vi "Initialize TX Transfer.vi"(7 "component name":string, 8 "error in":errorcluster, 9 "timeout (ms)":i32=1000 format="%.0f ms", 11 "Transfer Configuration in":refnum<class "Transfer Configuration.lvclass">) -> (0 "error out":errorcluster, 1 "buffer size":i32 format="%d bytes", 2 "timeout?":bool, 3 "transfer parameters":T1)   [LabVIEW 2020, in "RDMA.lvlib" / "RDMA Transceiver.lvclass"]
uses:
  RDMA Transceiver.lvclass
  DSF Core.lvlibp/Classes/Configuration/Core/Transfer/Transfer Configuration.lvclass
  Transfer Parameters.ctl
  Configuration/Tx Transfer/RDMA Transfer Tx Configuration.lvclass
  DSF Core.lvlibp/Classes/Configuration/Core/Core Configuration.lvclass
  <vilib>/rdma/rdma.llb/RDMA Direction.ctl
  <vilib>/rdma/rdma.llb/RDMA Configure Buffers U8.vi
  C:/git/fmussi-niveristand-data-sharing-framework-custom-device-plugins/Components/DSF Core.lvlibp/Classes/Configuration/Core/Core Configuration.lvclass
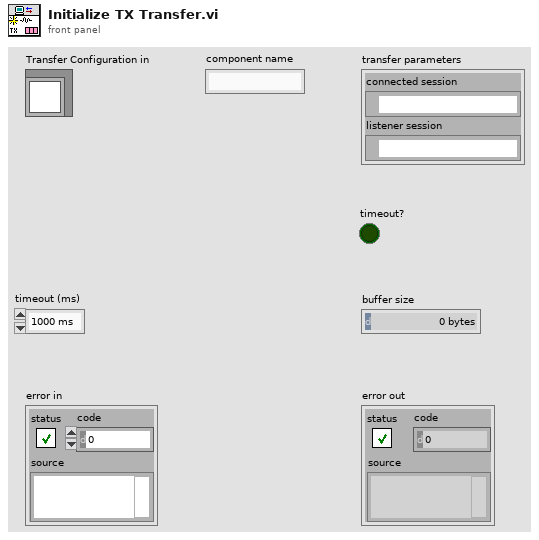
[diagram p1: front panel]
types:
  T1 = typedef "RDMA.lvlib/RDMA Transceiver.lvclass/Transfer Parameters.ctl" = cluster{"connected session":refnum<k21>, "listener session":refnum<k21>}
  T2 = typedef "DSF Core.lvlibp/DSF Settings Info.ctl" = cluster{"component":string, "values":cluster{"key":string, "value":string}[]}
  T3 = typedef "RDMA.lvlib/RDMA Transfer Tx Configuration.lvclass/Tx Transfer Settings.ctl" = cluster{"local address":u32, "local port":u16, "destination address":u32, "destination port":u16}
  T4 = typedef "RDMA Direction.ctl" = enum16{"Send", "Receive"}
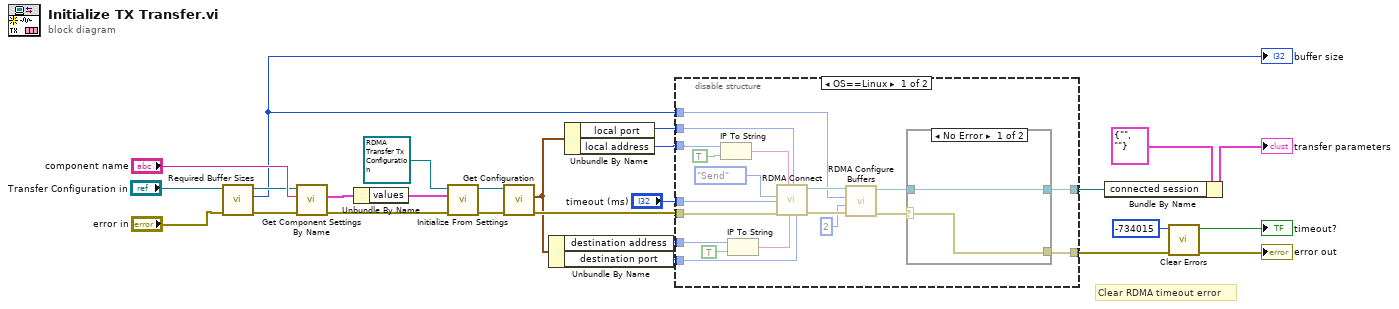
[diagram p0: block diagram]
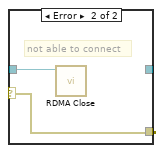
[diagram p2: hidden frame]
diagram:
  # "Clear RDMA timeout error"
  n1 = call-dynamic "Required Buffer Sizes.vi"("error in (no error)"="error in", "Transfer Configuration in"="Transfer Configuration in") -> ("error out"=w20:errorcluster, "engine size"=w19:u64, "Transfer Configuration out"=w21:refnum<class "Transfer Configuration.lvclass">)  [unwired: 6 in, 1 out]
  "buffer size" <- w19
  n2 = call "Get Component Settings By Name.vi"("error in (no error)"=w20, "component name"="component name", "Runtime Configuration in"=w21) -> ("error out"=w24:errorcluster, "component settings"=w23:T2)  [unwired: 6 in, 1 out]
  n3 = Unbundle By Name(w23) -> ("values"=w22:cluster{"key":string, "value":string}[])
  n4 = call-dynamic "Initialize From Settings.vi"("error in"=w24, "settings"=w22, "RDMA Tx Transfer Configuration in"=refnum<class "RDMA Transfer Tx Configuration.lvclass"> refnum ("UDP Tx Transfer Configuration in")) -> ("error out"=w17:errorcluster, "RDMA Tx Transfer Configuration out"=w16:refnum<class "RDMA Transfer Tx Configuration.lvclass">)  [unwired: 7 in]
  n5 = call "Get Configuration.vi"("error in"=w17, "RDMA Transfer Tx Configuration in"=w16) -> ("error out"=w15:errorcluster, "transfer settings"=w13:T3)  [unwired: 7 in, 1 out]
  n6 = Unbundle By Name(w13) -> ("destination address"=w11:u32, "destination port"=w12:u16)
  n7 = Unbundle By Name(w13) -> ("local port"=w9:u16, "local address"=w10:u32)
  n8 = disable-structure shown="OS==Linux" {
    disable-tunnel: [w35 w50] -> w1
    disable-tunnel: w19 -> [w32 _]
    disable-tunnel: w11 -> [w45 _]
    disable-tunnel: w12 -> [w44 _]
    disable-tunnel: w15 -> [w43 w50]
    disable-tunnel: w9 -> [w36 _]
    disable-tunnel: w10 -> [w37 _]
    disable-tunnel: [w28 _] -> w6
    disable-tunnel: "timeout (ms)" -> [w27 _]
    frame condition #0 {
      n9 = IP To String(1:TRUE ("dot notation? (F)"), 2:w37) -> (0:w40:string)
      n10 = IP To String(1:TRUE ("dot notation? (F)"), 2:w45) -> (0:w39:string)
      n11 = call <vilib>:"RDMA Connect.vi"("remote port"=w44, "local port"=w36, "remote address"=w39, "local address"=w40, "error in"=w43, "timeout (ms)"=w27, "direction"=RDMA_Direction."Send") -> ("error out"=w33:errorcluster, "rdma session"=w34:refnum<k21>)  [unwired: 3 in]
      n12 = call-poly <vilib>:"RDMA Configure Buffers.vi"("error in"=w33, "max concurrent transactions"=u64 2, "max transaction size"=w32, "rdma session in"=w34) -> ("error out"=w29:errorcluster, "rdma session out"=w30:refnum<k21>)  [unwired: 6 in]
      n13 = case shown="No Error" w29 {
        selector: w29 -> [w47 w48]
        tunnel: [w47 w48] -> w35
        tunnel: w30 -> [w46 w49]
        tunnel: [w46 _] -> w28
        frame No Error {
        }
        frame Error {
          # "not able to connect"
          n14 = call <vilib>:"RDMA Close.vi"("rdma session"=w49) -> ()  [unwired: 10 in, 1 out]
        }
      }
    }
    frame condition #1 (active) {
    }
  }
  n15 = Bundle By Name(cluster=T1 {"connected session"="", "listener session"=""} ("Transfer Tx"), "connected session"=w6) -> (→"transfer parameters":T1)
  n16 = call <vilib>:"Clear Errors.vi"("error in (no error)"=w1, "specific error code to clear (0: all)"=-734015) -> ("error out"=→"error out":errorcluster, "specific error cleared?"=→"timeout?":bool)  [unwired: 4 in]
